vi "Guests Manager.vi"() -> ()   [LabVIEW 2023]
panel:
  in  "Food Order 3":bool
  in  "Bill Details 2":string
  in  "Bill Details":string
  in  "Guest Contact Number":string
  in  "Primary Guest Name":string
  in  "Room Number":u16(ring) items=["305"]
  in  "Food Order 2":bool
  out "Remove Button 2":bool
  out "Add Button 2":bool
  out "Remove Button":bool
  out "Add Button":bool
  in  "Children":dbl
  in  "Adults":dbl
  in  "Back":bool
  in  "Room Number":u16(ring) items=["305"]
  in  "Room Size":u16(ring) items=["Suite (Non-AC)"]
  in  "Guest Contact Number":string
  in  "Primary Guest Name":string
  # "Guest Check-Out"
  # "Guest Check-In"
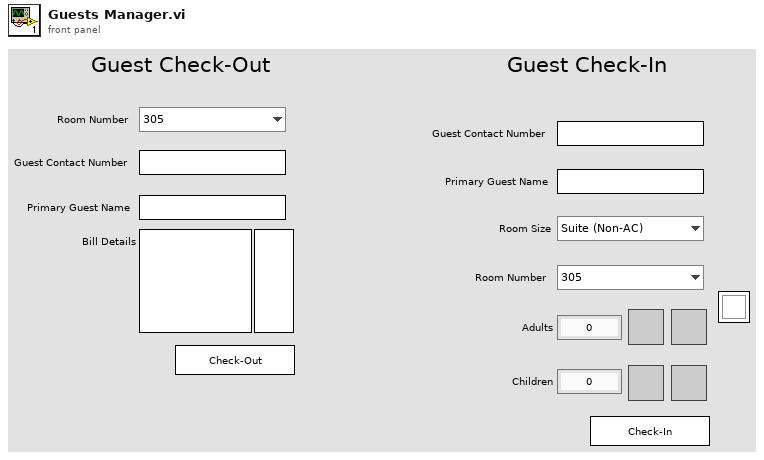
[diagram p1: front panel]
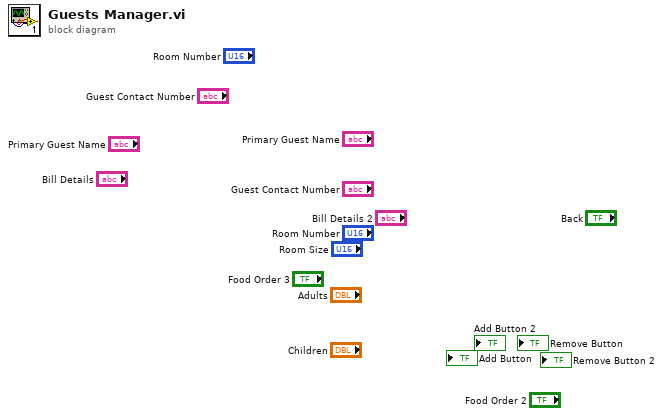
[diagram p0: block diagram]
diagram:
